vi "test Encode and Decode - Discretes and Float.vi"(8 "error in (no error)":errorcluster, 11 "TestCase in":refnum<class "AIM ARINC 664 EncodeDecode.lvclass">) -> (0 "error out":errorcluster, 3 "TestCase out":refnum<class "AIM ARINC 664 EncodeDecode.lvclass">)   [LabVIEW 2020, in "AIM ARINC 664 EncodeDecode.lvclass"]
uses:
  AIM ARINC 664 EncodeDecode.lvclass
  Shared/Encoding (Arinc664).ctl
  <vilib>/addons/_JKI Toolkits/VI Tester/TestCase.llb/TestCase.lvclass
  C:/Program Files/National Instruments/LabVIEW 2024/vi.lib/addons/_JKI Toolkits/VI Tester/TestCase.llb/TestCase.lvclass
panel:
  out "Values out":dbl[](array[numeric])
  in  "number of floats":i32=2
  out "index of first error":i32
  out "Parameters":T2(array[cluster]) {"encoding" items=["BNR", "BCD", "Discrete", "Signed_32", "Signed_64", "Float_32", "Float_64", "Opaque"]}
  in  "number of discretes":i32=8
  out "Result array out":bool[](array[boolean])
  out "Values in":dbl[](array[numeric])
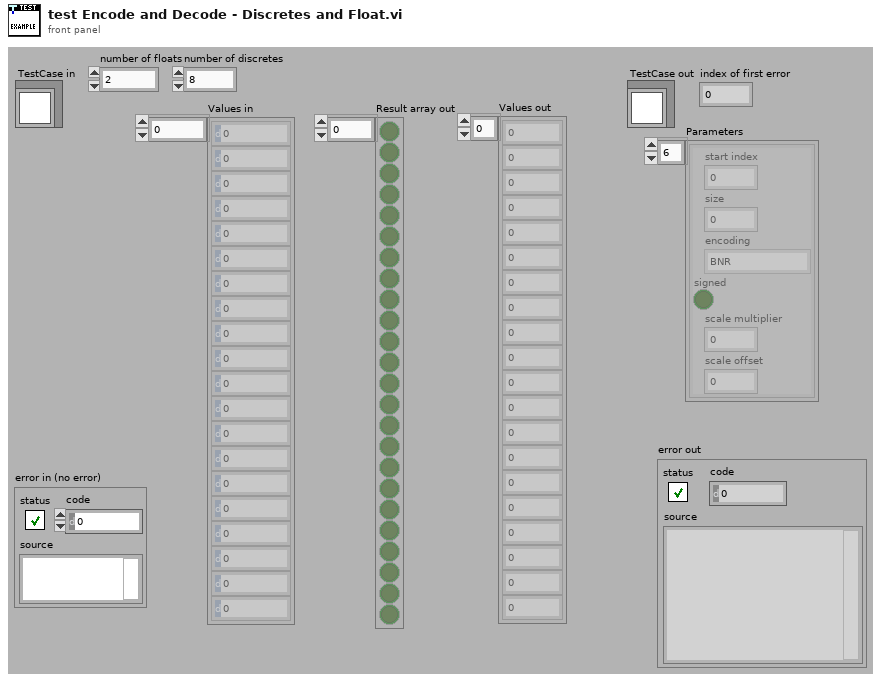
[diagram p1: front panel]
types:
  T1 = typedef "Encoding (Arinc664).ctl" = u16
  T2 = cluster{"start index":i32, "size":i32, "encoding":T1, "signed":bool, "scale multiplier":dbl, "scale offset":dbl}[]
  T3 = cluster{"start index":i32, "size":i32, "encoding":T1, "signed":bool, "scale multiplier":dbl, "scale offset":dbl}
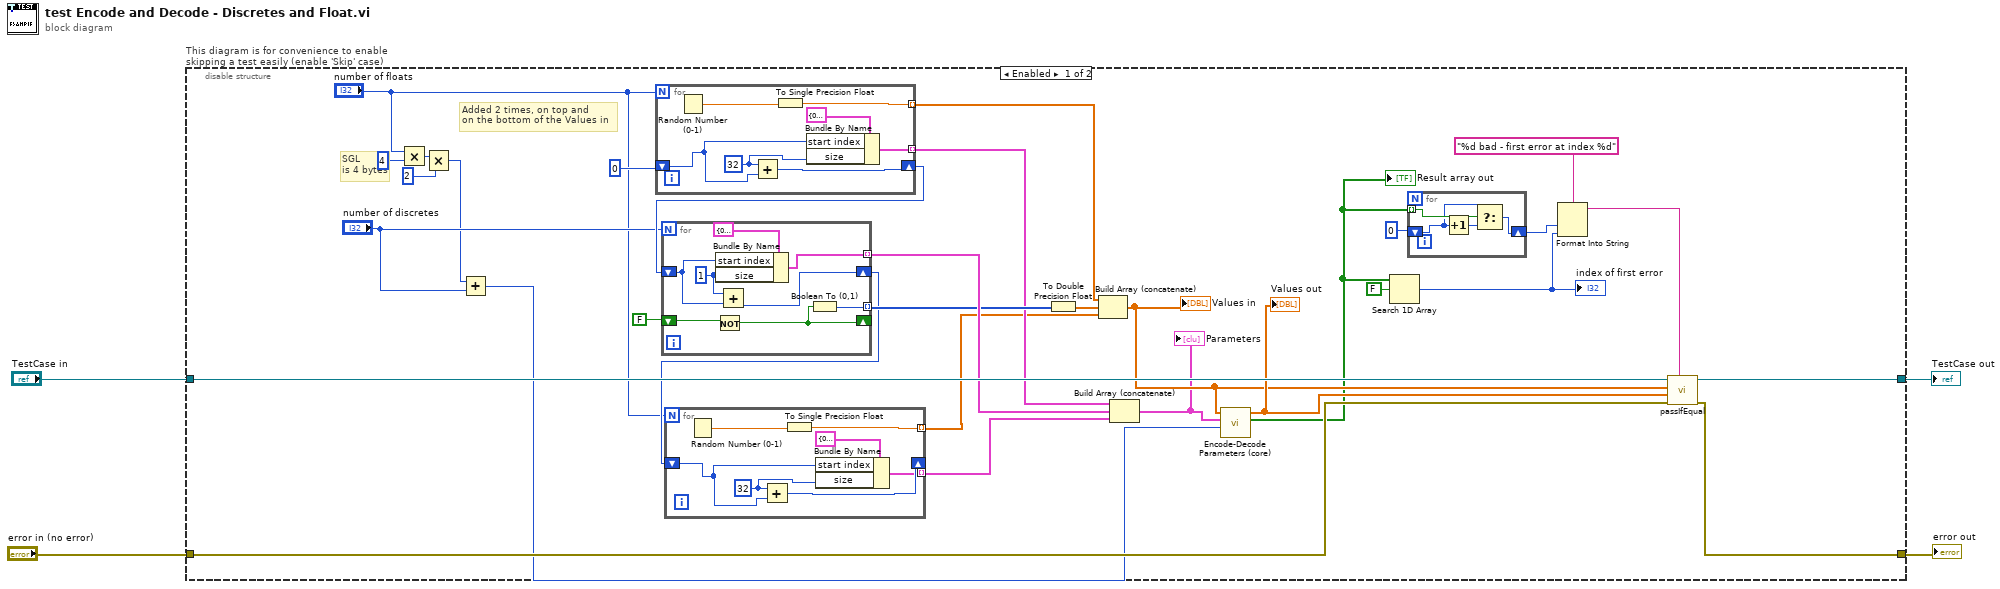
[diagram p0: block diagram]
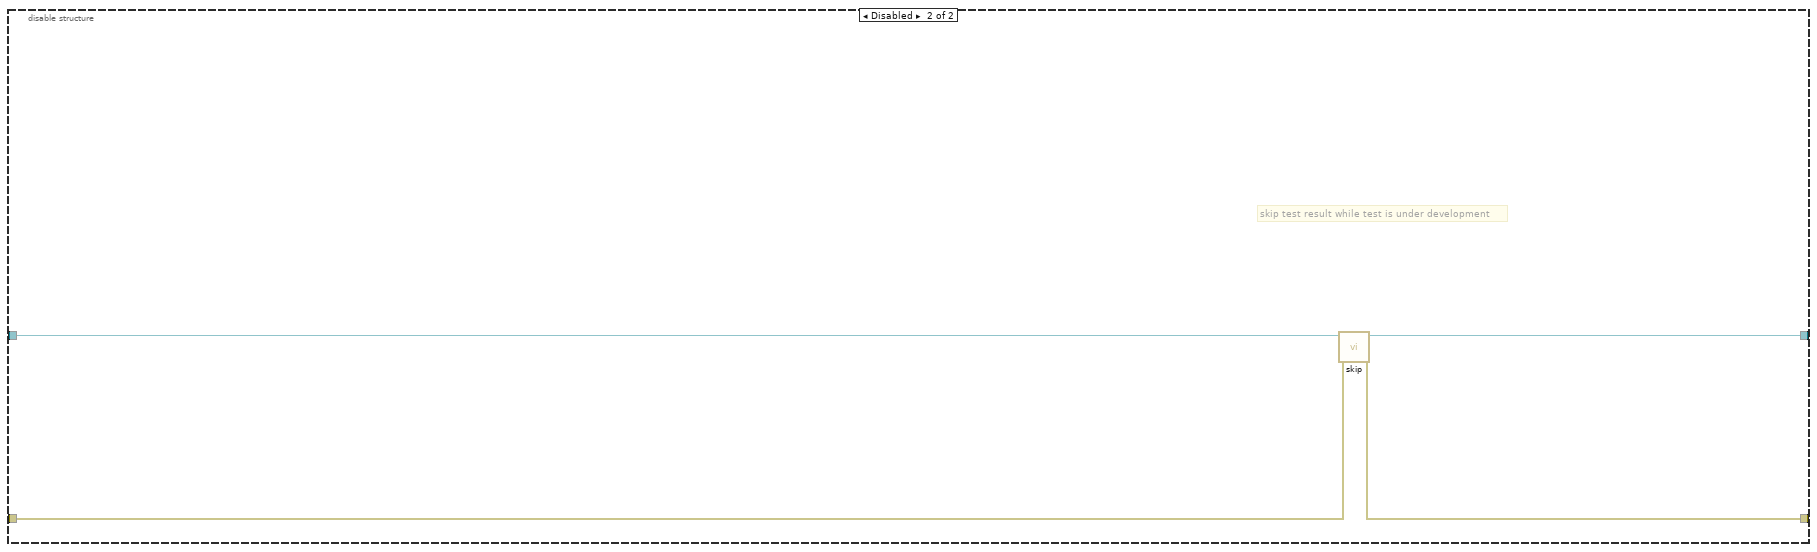
[diagram p2: hidden frame]
diagram:
  n1 = disable-structure "This diagram is for convenience to enable skipping a test easily (enable 'Skip' case)" shown="Enabled" {
    disable-tunnel: "TestCase in" -> [w36 w66]
    disable-tunnel: [w33 w64] -> w1
    disable-tunnel: [w34 w65] -> w3
    disable-tunnel: "error in (no error)" -> [w35 w63]
    frame Enabled {
      # "SGL\nis 4 bytes"
      # "Added 2 times, on top and \non the bottom of the Values in"
      n2 = Multiply(x="number of floats", y=4) -> (x*y=w15:i32)
      n3 = Multiply(x=w15, y=2) -> (x*y=w11:i32)
      n4 = Add(x=w11, y="number of discretes") -> (x+y=w13:i32)
      n5 = for {
        N: "number of floats" -> [_]
        tunnel: [w37] -> w12 mode=indexing
        shift-right: [w40] -> w23
        shift-left: 0 -> [w41]
        tunnel: [w38] -> w9 mode=indexing
        w39 = 32 ("x")
        n6 = Random Number (0-1)() -> (number: 0 to 1=w43:dbl)
        n7 = Add(x=w39, y=w41) -> (x+y=w40:i32)
        n8 = To Single Precision Float(number=w43) -> (single precision float=w37:sgl)
        n9 = Bundle By Name(cluster=T3 {"start index"=0, "size"=64, "encoding"=5, "signed"=TRUE, "scale multiplier"=1.0, "scale offset"=0.0} ("Parameters 2"), "start index"=w41, "size"=w39) -> (w38:T3)
      }
      n10 = for {
        N: "number of discretes" -> [_]
        shift-right: [w49] -> _
        shift-left: FALSE -> [w50]
        tunnel: [w48] -> w29 mode=indexing
        tunnel: [w47] -> w30 mode=indexing
        shift-right: [w44] -> w8
        shift-left: w23 -> [w45]
        w46 = 1 ("size")
        n11 = Not(x=w50) -> (.not. x?=w49:bool)
        n12 = Bundle By Name(cluster=T3 {"start index"=0, "size"=64, "encoding"=2, "signed"=TRUE, "scale multiplier"=1.0, "scale offset"=0.0} ("Parameters 2"), "start index"=w45, "size"=w46) -> (w47:T3)
        n13 = Add(x=w46, y=w45) -> (x+y=w44:i32)
        n14 = Boolean To (0,1)(Boolean=w49) -> (0, 1=w48:i16)
      }
      n15 = for {
        N: "number of floats" -> [_]
        tunnel: [w56] -> w6 mode=indexing
        shift-right: [w59] -> _
        shift-left: w8 -> [w60]
        tunnel: [w57] -> w7 mode=indexing
        w58 = 32 ("x")
        n16 = Random Number (0-1)() -> (number: 0 to 1=w62:dbl)
        n17 = Add(x=w58, y=w60) -> (x+y=w59:i32)
        n18 = To Single Precision Float(number=w62) -> (single precision float=w56:sgl)
        n19 = Bundle By Name(cluster=T3 {"start index"=0, "size"=64, "encoding"=5, "signed"=TRUE, "scale multiplier"=1.0, "scale offset"=0.0} ("Parameters 2"), "start index"=w60, "size"=w58) -> (w57:T3)
      }
      n20 = To Double Precision Float(number=w29) -> (double precision float=w28:dbl[])
      n21 = Build Array (concatenate)(w12, w28, w6) -> (w25:dbl[])
      "Values in" <- w25
      n22 = Build Array (concatenate)(w9, w30, w7) -> (w24:T2)
      "Parameters" <- w24
      n23 = call "Encode-Decode Parameters (core).vi"("Payload size - bytes"=w13, "Parameters"=w24, "Values in"=w25) -> ("Result array out"=w22:bool[], "Values out"=w32:dbl[])  [unwired: 7 in]
      "Result array out" <- w22
      "Values out" <- w32
      n24 = Search 1D Array(1D array=w22, element=FALSE) -> (index of element=w19:i32)  [unwired: 1 in]
      "index of first error" <- w19
      n25 = for {
        tunnel: w22 -> [w55] mode=indexing
        shift-right: [w52] -> w20
        shift-left: 0 -> [w53]
        n26 = Increment(x=w53) -> (x+1=w54:i32)
        n27 = Select(t=w53, s=w55, f=w54) -> (s? t:f=w52:i32)
      }
      n28 = Format Into String(format string="%d bad - first error at index %d", w20, w19) -> (resulting string=w17:string)  [unwired: 2 in, 1 out]
      n29 = call-dynamic "passIfEqual.vi"("custom report message (\"\")"=w17, "error in (no error)"=w35, "y"=w32, "x"=w25, "TestCase in"=w36) -> ("error out"=w34:errorcluster, "TestCase out"=w33:refnum<class "AIM ARINC 664 EncodeDecode.lvclass">)  [unwired: 5 in]
    }
    frame Disabled {
      # "skip test result while test is under development"
      n30 = call <vilib>:"skip.vi"("error in (no error)"=w63, "TestCase in"=w66) -> ("error out"=w65:errorcluster, "TestCase out"=w64:refnum<class "AIM ARINC 664 EncodeDecode.lvclass">)  [unwired: 8 in]
    }
  }
  "error out" <- w3
  "TestCase out" <- w1
